vi "LauftextUhr.vi"(1 "Intensity 0-100":dbl(knob) min=0.0 max=100.0 step=1.0 scale=0.0..100.0, 2 "VISA resource name":refnum<visa-resource-name>) -> (0 "VISA resource name 2":refnum<visa-resource-name>)   [LabVIEW 2021]
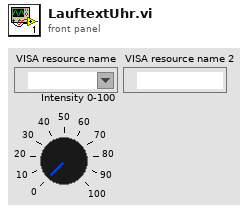
[diagram p1: front panel]
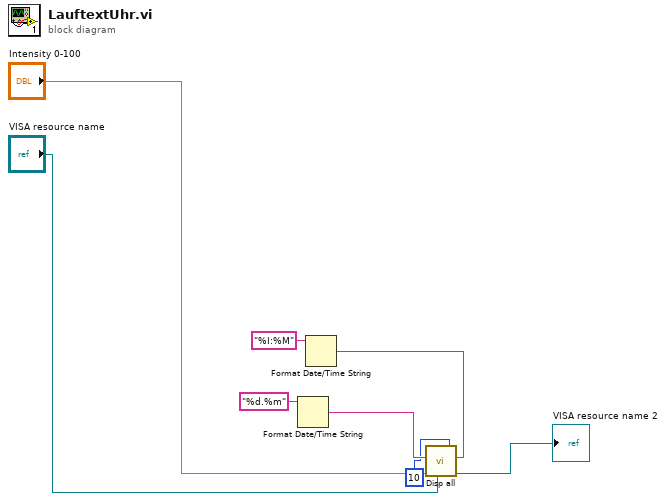
[diagram p0: block diagram]
diagram:
  n1 = Format Date/Time String(time format string (%c)="%d.%m") -> (date/time string=w8:string)  [unwired: 2 in]
  n2 = Format Date/Time String(time format string (%c)="%I:%M") -> (date/time string=w7:string)  [unwired: 2 in]
  n3 = call "Disp all.vi"("Time"=w7, "milliseconds to wait betweeen frames"=u32 10, "VISA resource name"="VISA resource name", "Intensity 0-100"="Intensity 0-100", "Date"=w8) -> ("VISA resource name 2"=→"VISA resource name 2":refnum<visa-resource-name>)  [unwired: 4 in]
